vi "脉冲生成_基于时间_有限.vi"() -> ()   [LabVIEW 2013]
uses:
  <userlib>/ArtDAQ/_SubVI/ArtDAQ_CreateCOPulseChanTime.vi
  <userlib>/ArtDAQ/_SubVI/ArtDAQ_CfgImplicitTiming.vi
  <userlib>/ArtDAQ/_SubVI/ArtDAQ_CfgDigEdgeStartTrig.vi
panel:
  in  "触发模式":enum32{"No Trigger", "DigStartTrig"}(tab)
  in  "触发边沿":i32(ring)=10280 items=["上升"=10280, "下降"=10171]
  in  "触发源":string(combo)="/Dev1/PFI1"
  in  "每通道采样点数":i32=1000
  in  "停止":bool
  in  "计数器":string="Dev1/ctr0"
  in  "高电平时间":dbl=0.01 format="%0.6f"
  in  "低电平时间":dbl=0.01 format="%0.6f"
  out "错误输出":errorcluster
  # "通道属性"
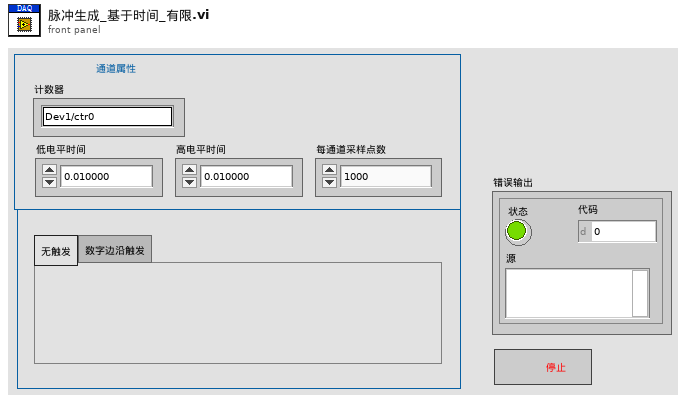
[diagram p1: front panel]
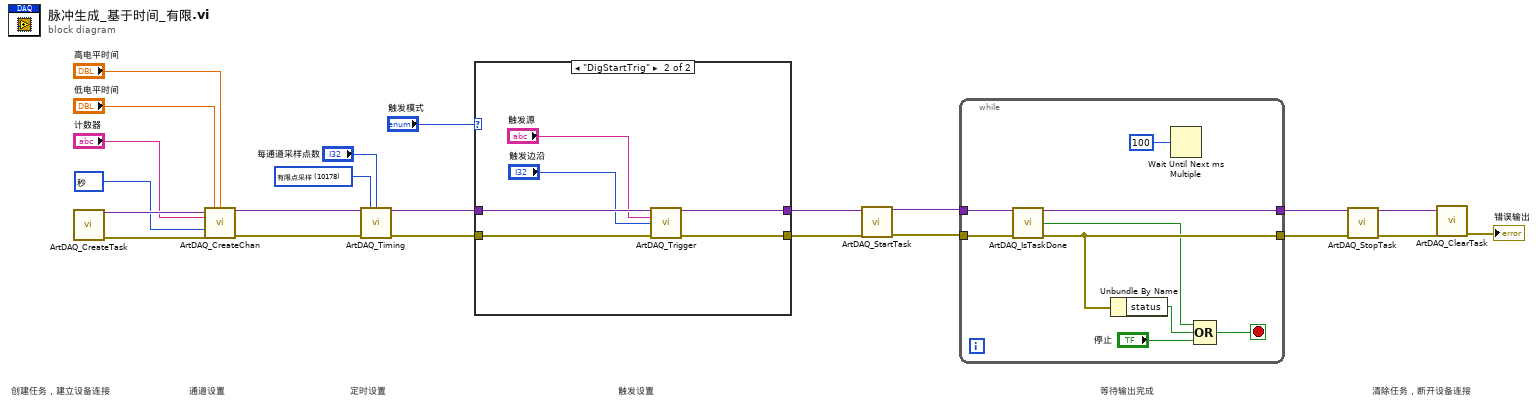
[diagram p0: block diagram]
diagram:
  w1 = 10364 items=["秒"=10364] ("Units")
  w10 = 10178 items=["有限点采样"=10178, "连续采样"=10123] ("SampleMode")
  # "清除任务，断开设备连接"
  # "等待输出完成"
  # "触发设置"
  # "定时设置"
  # "通道设置"
  # "创建任务，建立设备连接"
  n1 = call <userlib>:"ArtDAQ_CreateTask.vi"() -> ("任务句柄"=w22:variant, "错误输出"=w21:errorcluster)  [unwired: 14 in]
  n2 = call-poly <userlib>:"ArtDAQ_CreateChan.vi"("任务句柄"=w22, "低时间"="低电平时间", "高时间"="高电平时间", "计数器"="计数器", "单位"=w1, "错误输入"=w21) -> ("任务句柄"=w12:variant, "错误输出"=w11:errorcluster)  [unwired: 8 in]
  n3 = call-poly <userlib>:"ArtDAQ_Timing.vi"("任务句柄"=w12, "采样模式"=w10, "每通道采样数"="每通道采样点数", "错误输入"=w11) -> ("任务句柄"=w7:variant, "错误输出"=w6:errorcluster)  [unwired: 10 in]
  n4 = case shown="\"DigStartTrig\"" "触发模式" {
    tunnel: w7 -> [w24 w30]
    tunnel: [w24 w29] -> w5
    tunnel: [w23 w28] -> w3
    tunnel: w6 -> [w23 w27]
    frame "No Trigger", Default {
    }
    frame "DigStartTrig" {
      n5 = call-poly <userlib>:"ArtDAQ_Trigger.vi"("任务句柄"=w30, "触发源"="触发源", "边沿"="触发边沿", "错误输入"=w27) -> ("任务句柄"=w29:variant, "错误输出"=w28:errorcluster)  [unwired: 10 in]
    }
  }
  n6 = call <userlib>:"ArtDAQ_StartTask.vi"("任务句柄"=w5, "错误输入"=w3) -> ("任务句柄"=w4:variant, "错误输出"=w2:errorcluster)  [unwired: 12 in]
  n7 = while {
    tunnel: [w39] -> w19
    tunnel: [w38] -> w17
    tunnel: w4 -> [w35]
    tunnel: w2 -> [w34]
    stop <- w33 stop-if-true
    n8 = call <userlib>:"ArtDAQ_IsTaskDone.vi"("任务句柄"=w35, "错误输入"=w34) -> ("任务句柄"=w39:variant, "完成任务？"=w31:bool, "错误输出"=w38:errorcluster)  [unwired: 11 in]
    n9 = Unbundle By Name(w38) -> ("status"=w37:bool)
    n10 = Wait Until Next ms Multiple(millisecond multiple=u32 100 ("毫秒倍数")) -> ()  [unwired: 1 out]
    n11 = Compound Arithmetic op=OR(w31, w37, "停止") -> (w33:bool)
  }
  n12 = call <userlib>:"ArtDAQ_StopTask.vi"("任务句柄"=w19, "错误输入"=w17) -> ("任务句柄"=w18:variant, "错误输出"=w16:errorcluster)  [unwired: 12 in]
  n13 = call <userlib>:"ArtDAQ_ClearTask.vi"("任务句柄"=w18, "错误输入"=w16) -> ("错误输出"=→"错误输出":errorcluster)  [unwired: 13 in]
